vi "Memory.Pointer.Deallocate.vi"(7 "allocation limit (2^31: 2GiB)":u64=2147483647 format="%08x bytes", 8 "error in (no error)":errorcluster, 10 "size":u64 format="%d bytes", 11 "Pointer in":refnum<class "Memory.Pointer.Void.lvclass">) -> (0 "error out":errorcluster, 2 "allocated size":i64=2147483647 format="%08x bytes", 3 "Pointer out":refnum<class "Memory.Pointer.Void.lvclass">)   [LabVIEW 2016, in "LabVIEW Memory Manager.lvlib" / "Memory.Pointer.Void.lvclass"]
uses:
  Memory.Pointer.Void.lvclass
  Memory.Pointer.Void.lvclass/Memory.Pointer.Void.ctl
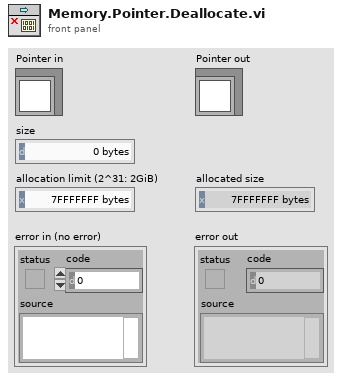
[diagram p1: front panel]
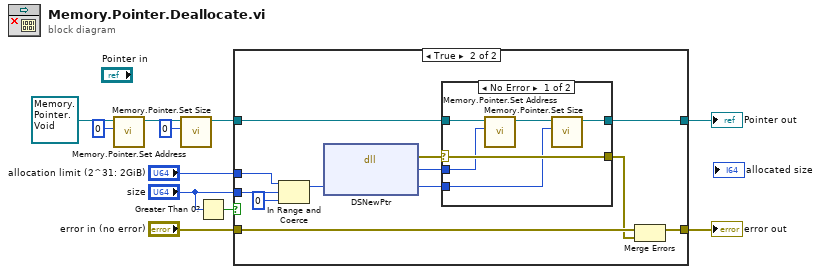
[diagram p0: block diagram]
diagram:
  n1 = call "Memory.Pointer.Set Address.vi"("address"=u64 0, "Pointer in"=refnum<class "Memory.Pointer.Void.lvclass"> refnum ("LabVIEW Memory Manager.lvlib:Pointer")) -> ("Pointer out"=w5:refnum<class "Memory.Pointer.Void.lvclass">)  [unwired: 8 in, 1 out]
  n2 = call "Memory.Pointer.Set Size.vi"("size"=u64 0, "Pointer in"=w5) -> ("Pointer out"=w2:refnum<class "Memory.Pointer.Void.lvclass">)  [unwired: 8 in, 1 out]
  n3 = Greater Than 0?(x="size") -> (x > 0?=w8:bool)
  n4 = case shown="True" w8 {
    tunnel: w2 -> [w12 w14]
    tunnel: "size" -> [_ w17]
    tunnel: [w12 w24] -> w11
    tunnel: "error in (no error)" -> [w13 w21]
    tunnel: [w13 w20] -> w9
    tunnel: "allocation limit (2^31: 2GiB)" -> [_ w18]
    frame False {
    }
    frame True {
      n5 = In Range and Coerce(upper limit=w18, x=w17, lower limit=u64 0) -> (coerced(x)=w16:u64)  [unwired: 1 out]
      n6 = dll-call lib="LabVIEW" fn="DSNewPtr"("size"=w16) -> (error out=w22:errorcluster, "pointer"=w25:u64, "size"=w23:u64)  [unwired: 3 in, 1 out]
      n7 = case shown="No Error" w22 {
        selector: w22 -> [w28 w33]
        tunnel: w14 -> [w31 w32]
        tunnel: w25 -> [w27 _]
        tunnel: [w29 w32] -> w24
        tunnel: w23 -> [w26 _]
        tunnel: [w28 w33] -> w15
        frame No Error {
          n8 = call "Memory.Pointer.Set Address.vi"("address"=w27, "Pointer in"=w31) -> ("Pointer out"=w30:refnum<class "Memory.Pointer.Void.lvclass">)  [unwired: 8 in, 1 out]
          n9 = call "Memory.Pointer.Set Size.vi"("size"=w26, "Pointer in"=w30) -> ("Pointer out"=w29:refnum<class "Memory.Pointer.Void.lvclass">)  [unwired: 8 in, 1 out]
        }
        frame Error {
        }
      }
      n10 = Merge Errors(w21, w15) -> (w20:errorcluster)
    }
  }
  "error out" <- w9
  "Pointer out" <- w11
